vi "Threshold.vi"(1 "Threshold":dbl=0.5, 2 "Normalised Time Serie [\\]":dbl[](array[numeric])) -> (0 "Thresholded Time Serie [\\]":dbl[](array[numeric]))   [LabVIEW 2023]
doc: "This simple VI is aimed at set to 0 the values of the normalised input time serie in input whose value is below the threshold.\nInputs:\n- Normalised Time Serie\nOutputs:\n- Masked Time Serie"
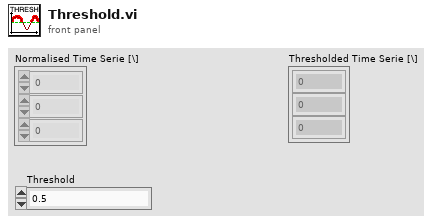
[diagram p1: front panel]
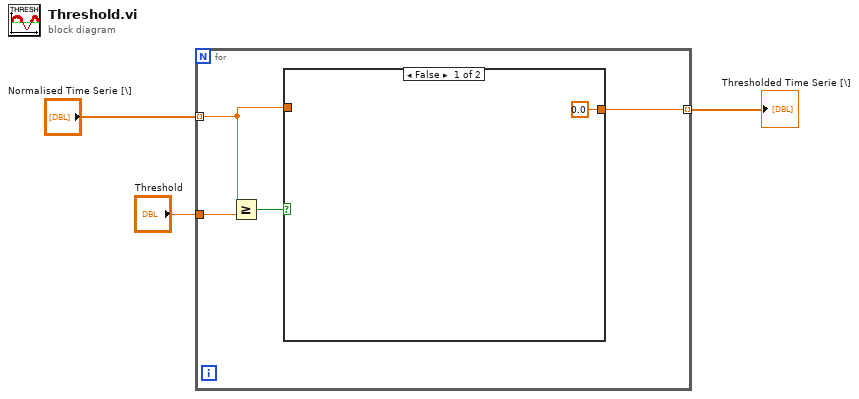
[diagram p0: block diagram]
diagram:
  n1 = for {
    tunnel: "Normalised Time Serie [\\]" -> [w6] mode=indexing
    tunnel: [w5] -> w2 mode=indexing
    tunnel: "Threshold" -> [w4]
    n2 = Greater Or Equal?(x=w6, y=w4) -> (x >= y?=w7:bool)
    n3 = case shown="False" w7 {
      tunnel: [0.0 ("Numeric") w9] -> w5
      tunnel: w6 -> [_ w9]
      frame False {
      }
      frame True {
      }
    }
  }
  "Thresholded Time Serie [\\]" <- w2
